vi "Config to String.vi"(8 "error in (no error)":errorcluster, 11 "DSF Configuration Reference in":T1) -> (0 "error out":errorcluster, 2 "String":string, 3 "DSF Configuration Reference out":T1)   [LabVIEW 2017, in "DSF Configuration API.lvlib"]
uses:
  DSF Configuration API.lvlib
  Controls/Session/DSF Configuration Reference.ctl
  Controls/Session/Config Data.ctl
  Controls/DSF File Format/DSF Config.ctl
  Public/Controls/Version Info.ctl
  Controls/DSF File Format/DSF Plugin.ctl
  Public/Controls/DSF Plugin Info.ctl
  Public/Controls/DSF Timing Info.ctl
  Controls/DSF File Format/DSF Group.ctl
  Public/Controls/DSF Group Info.ctl
  Controls/DSF File Format/DSF Transfer.ctl
  Public/Controls/DSF Transfer Info.ctl
  Controls/DSF File Format/DSF Channel.ctl
  Public/Controls/DSF Channel Info.ctl
  Controls/DSF File Format/DSF Settings.ctl
  Public/Controls/DSF Settings Info.ctl
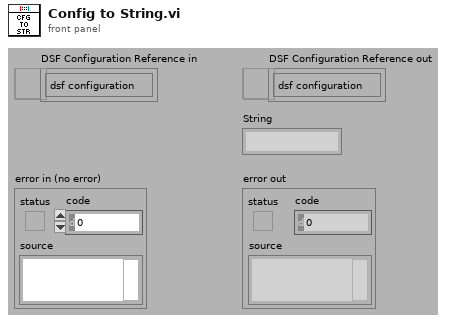
[diagram p1: front panel]
types:
  T1 = typedef "DSF Configuration API.lvlib/DSF Configuration Reference.ctl" = refnum<data-value>
  T2 = typedef "DSF Configuration API.lvlib/Config Data.ctl" = cluster{"dsf configuration":T3, "path":path, "dirty":bool}
  T3 = typedef "DSF Configuration API.lvlib/DSF Config.ctl" = cluster{"dsfversion":T4, "version":T4, "plugins":T5[], "groups":T8[], "transfers":T10[], "channels":T12[], "settings":T14[]}
  T4 = typedef "DSF Configuration API.lvlib/Version Info.ctl" = cluster{"major":u32, "minor":u32, "fix":u32, "build":string}
  T5 = typedef "DSF Configuration API.lvlib/DSF Plugin.ctl" = cluster{"id":string, "values":T6}
  T6 = typedef "DSF Configuration API.lvlib/DSF Plugin Info.ctl" = cluster{"type":string, "timing":T7, "group ids":string[], "settings id":string}
  T7 = typedef "DSF Configuration API.lvlib/DSF Timing Info.ctl" = cluster{"priority":i32, "decimation":i32, "offset":i32}
  T8 = typedef "DSF Configuration API.lvlib/DSF Group.ctl" = cluster{"id":string, "values":T9}
  T9 = typedef "DSF Configuration API.lvlib/DSF Group Info.ctl" = cluster{"direction":i32, "timing":T7, "transfer ids":string[], "settings id":string}
  T10 = typedef "DSF Configuration API.lvlib/DSF Transfer.ctl" = cluster{"id":string, "values":T11}
  T11 = typedef "DSF Configuration API.lvlib/DSF Transfer Info.ctl" = cluster{"byte order":i32, "channel ids":string[], "settings id":string}
  T12 = typedef "DSF Configuration API.lvlib/DSF Channel.ctl" = cluster{"id":string, "values":T13}
  T13 = typedef "DSF Configuration API.lvlib/DSF Channel Info.ctl" = cluster{"count":i32, "offset":i32, "data type":i32, "resource path":string, "settings id":string}
  T14 = typedef "DSF Configuration API.lvlib/DSF Settings.ctl" = cluster{"id":string, "values":T15}
  T15 = typedef "DSF Configuration API.lvlib/DSF Settings Info.ctl" = cluster{"key":string, "value":string}[]
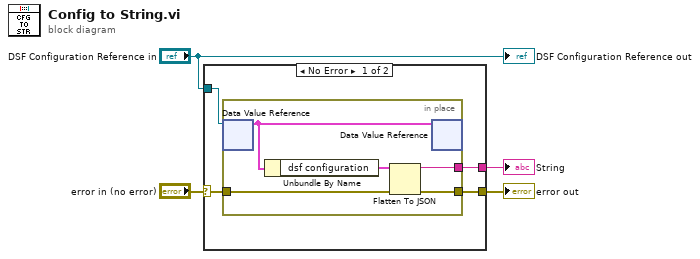
[diagram p0: block diagram]
diagram:
  n1 = case shown="No Error" "error in (no error)" {
    selector: "error in (no error)" -> [w7 w14]
    tunnel: "DSF Configuration Reference in" -> [w5 _]
    tunnel: [w8 _] -> w4
    tunnel: [w6 w14] -> w2
    frame No Error {
      n2 = in-place {
        in-place-border: [w12] -> w8
        in-place-border: w7 -> [w11]
        in-place-border: [w10] -> w6
        n3 = in-place-dvr #1(w5) -> (w9:T2)  [unwired: 1 out]
        n4 = Unbundle By Name(w9) -> ("dsf configuration"=w13:T3)
        n5 = Flatten To JSON(anything=w13, error in (no error)=w11) -> (JSON string=w12:string, 11:w10:errorcluster)  [unwired: 1 in]
        n6 = in-place-dvr #1(w9) -> ()  [unwired: 2 out]
      }
    }
    frame Error {
    }
  }
  "error out" <- w2
  "String" <- w4
  "DSF Configuration Reference out" <- "DSF Configuration Reference in"
